vi "GetContextHelpInfo.vi"(0 "reference":refnum<class "AbstractNode.lvclass">, 1 "MousePos":T1 {"y" format="%.2f"; "x" format="%.2f"}, 5 "error in (no error)":errorcluster) -> (14 "reference out":refnum<class "AbstractNode.lvclass">, 15 "ContextHelpInfoExist":bool, 16 "ContextHelpInfo":variant, 19 "error out":errorcluster)   [LabVIEW 2016, in "AbstractNode.lvclass"]
doc: "GetContextHelpInfo"
uses:
  <resource>/Framework/Providers/Open_GDS/UML/AbstractNode_class/AbstractNode.lvclass
  <resource>/Framework/Providers/Open_GDS/UML/General/Point/Point Point2D.ctl
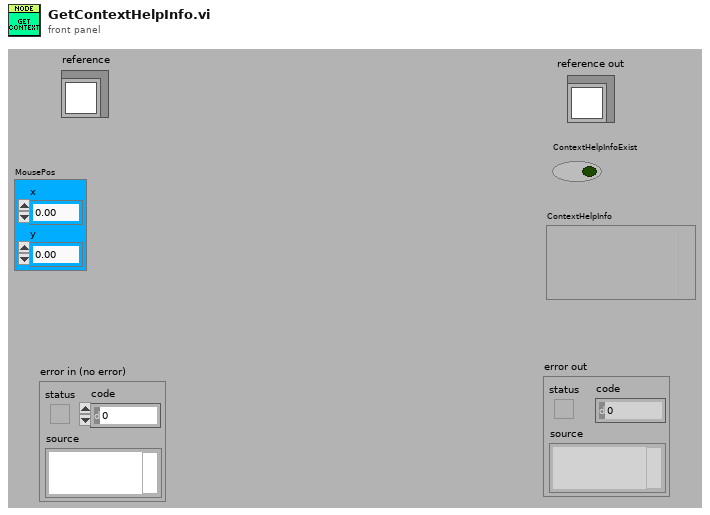
[diagram p1: front panel]
types:
  T1 = typedef "Point Point2D.ctl" = cluster{"x":dbl, "y":dbl}
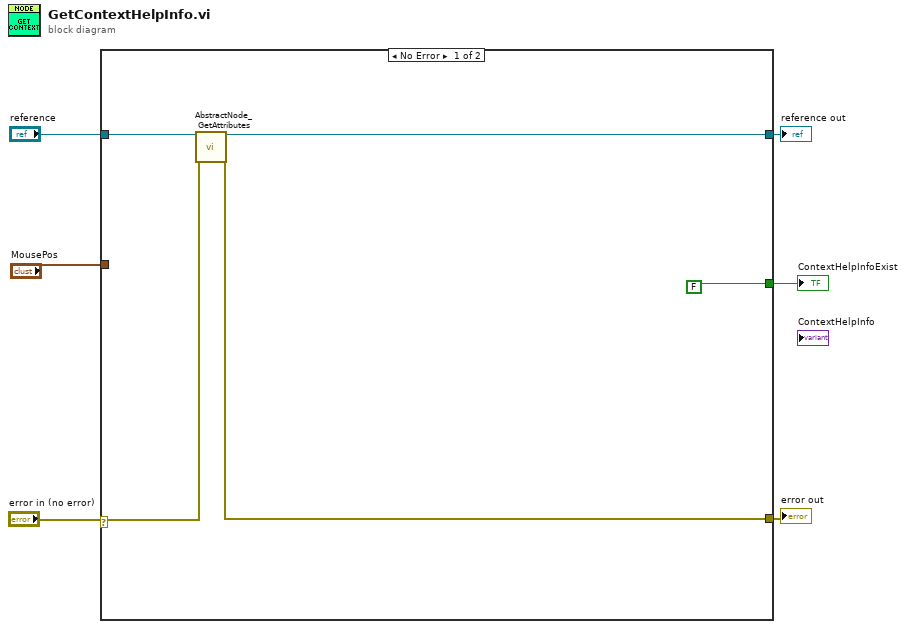
[diagram p0: block diagram]
diagram:
  n1 = case shown="No Error" "error in (no error)" {
    selector: "error in (no error)" -> [w8 w12]
    tunnel: "reference" -> [w11 w13]
    tunnel: [w10 w12] -> w5
    tunnel: [w9 w13] -> w4
    tunnel: [FALSE _] -> w2
    tunnel: "MousePos" -> [_ _]
    frame No Error {
      n2 = call <resource>:"AbstractNode_GetAttributes.vi"("reference in"=w11, "error in (no error)"=w8) -> ("reference out"=w9:refnum<class "AbstractNode.lvclass">, "error out"=w10:errorcluster)  [unwired: 1 in, 15 out]
    }
    frame Error {
    }
  }
  "reference out" <- w4
  "error out" <- w5
  "ContextHelpInfoExist" <- w2
